vi "Notify Monitor.vi"(8 "error in (no error)":errorcluster, 11 "Monitored Actor in":refnum<class "Monitored Actor.lvclass">) -> (0 "error out":errorcluster, 3 "Monitored Actor out":refnum<class "Monitored Actor.lvclass">)   [LabVIEW 2017, in "MGI-Monitored Actor Core.lvlib" / "Monitored Actor.lvclass"]
doc: "Notifies the actor monitor that a new actor has spawned\n\nCopyright: MGI 2016\nAuthor: Derek Trepanier"
uses:
  Monitored Actor.lvclass
  C:/Program Files (x86)/National Instruments/LabVIEW 2017/vi.lib/ActorFramework/Actor/Actor.lvclass
  <vilib>/ActorFramework/Actor/Actor.lvclass/Actor.ctl
  <vilib>/ActorFramework/Message Enqueuer/Message Enqueuer.lvclass/Message Enqueuer.ctl
  Monitored Actor.lvclass/Monitored Actor.ctl
  <vilib>/ActorFramework/Message Enqueuer/Init from Existing Queue.vi
  <vilib>/ActorFramework/Message Enqueuer/Message Enqueuer.lvclass
  <vilib>/ActorFramework/Actor/Actor.lvclass
  Actor Monitor/Actor Monitor Messages/Actor Launched Msg/Actor Launched Msg.lvclass
  Actor Monitor/Actor Monitor Messages/Update Label Msg/Update Label Msg.lvclass
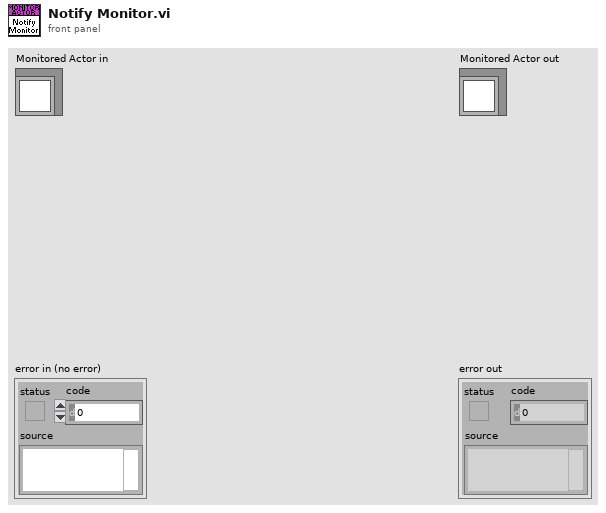
[diagram p1: front panel]
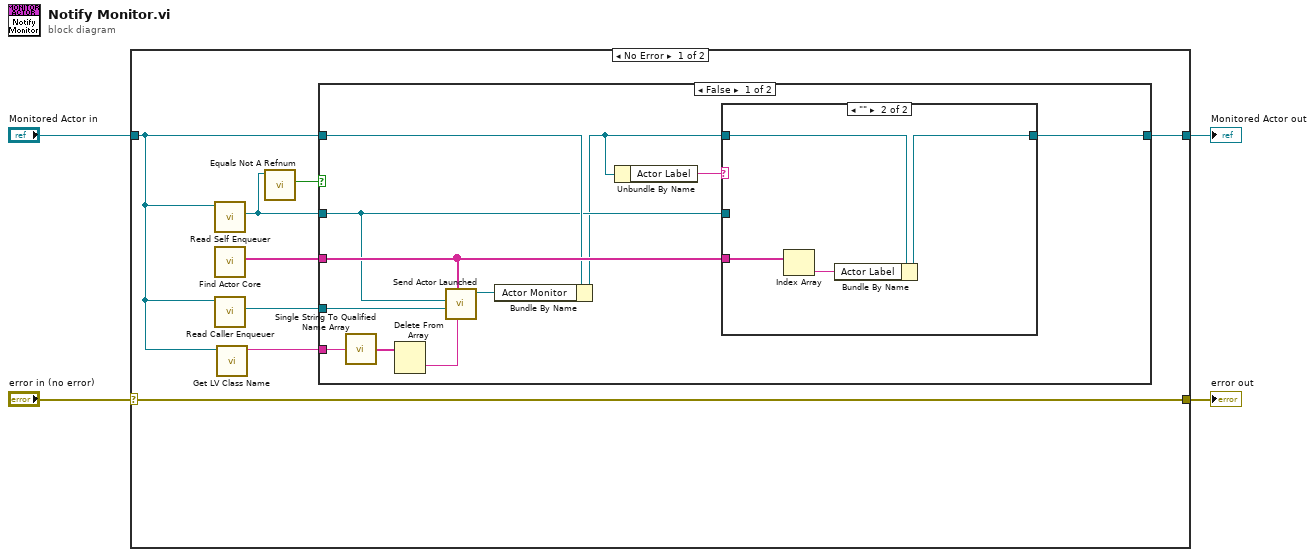
[diagram p0: block diagram]
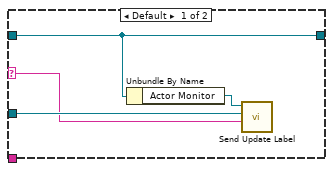
[diagram p2: hidden frame]
diagram:
  n1 = case shown="No Error" "error in (no error)" {
    selector: "error in (no error)" -> [w5 w34]
    tunnel: [w5 w34] -> w3
    tunnel: [w11 w33] -> w1
    tunnel: "Monitored Actor in" -> [w9 w33]
    frame No Error {
      n2 = call <vilib>:"Read Self Enqueuer.vi"("Actor"=w9) -> ("Self Enqueuer"=w7:refnum<class "Message Enqueuer.lvclass">)  [unwired: 10 in]
      n3 = call "Find Actor Core.vi"() -> ("Actor Cores"=w10:string[])  [unwired: 11 in]
      n4 = call <vilib>:"Read Caller Enqueuer.vi"("Actor"=w9) -> ("Caller Enqueuer"=w12:refnum<class "Message Enqueuer.lvclass">)  [unwired: 10 in]
      n5 = call <vilib>:"Get LV Class Name.vi"("object"=w9) -> ("class name"=w8:string)  [unwired: 9 in, 1 out]
      n6 = call <vilib>:"Equals Not A Refnum.vi"("Message Enqueuer"=w7) -> ("Not a refnum?"=w6:bool)  [unwired: 10 in]
      n7 = case shown="False" w6 {
        tunnel: w12 -> [w23 _]
        tunnel: [w22 w32] -> w11
        tunnel: w10 -> [w20 _]
        tunnel: w9 -> [w19 w32]
        tunnel: w8 -> [w17 _]
        tunnel: w7 -> [w18 _]
        frame False {
          n8 = call <vilib>:"Single String To Qualified Name Array.vi"("Fully Qualified String"=w17) -> ("Fully Qualified Array"=w16:string[])
          n9 = Delete From Array(array=w16) -> (deleted portion=w15:string)  [unwired: 2 in, 1 out]
          n10 = call "Send Actor Launched.vi"("Actor Type"=w15, "Actor Cores"=w20, "Actor's Caller Q"=w23, "Actor's Self Q"=w18) -> ("Message Enqueuer out"=w13:refnum<class "Message Enqueuer.lvclass">)  [unwired: 6 in, 1 out]
          n11 = Bundle By Name(cluster=w19, "Actor Monitor"=w13) -> (w14:refnum<class "Monitored Actor.lvclass">)
          n12 = Unbundle By Name(w14) -> ("Actor Label"=w21:string)
          n13 = case shown="\"\"" w21 {
            selector: w21 -> [w26 _]
            tunnel: w14 -> [w25 w31]
            tunnel: w18 -> [w27 _]
            tunnel: [w25 w30] -> w22
            tunnel: w20 -> [_ w29]
            frame Default {
              n14 = Unbundle By Name(w25) -> ("Actor Monitor"=w24:refnum<class "Message Enqueuer.lvclass">)
              n15 = call "Send Update Label.vi"("Actor's Label"=w26, "Actor's Self Q"=w27, "Message Enqueuer in"=w24) -> ()  [unwired: 7 in, 2 out]
            }
            frame "" {
              n16 = Index Array(array=w29) -> (element=w28:string)  [unwired: 1 in]
              n17 = Bundle By Name(cluster=w31, "Actor Label"=w28) -> (w30:refnum<class "Monitored Actor.lvclass">)
            }
          }
        }
        frame True {
        }
      }
    }
    frame Error {
    }
  }
  "error out" <- w3
  "Monitored Actor out" <- w1
